vi "testNewArduino.vi"() -> ()   [LabVIEW 2012]
panel:
  in  "valve value":bool
  in  "valve id":i32
  in  "VISA resource":refnum<visa-resource-name>="COM3"
  in  "speed":i32
  in  "Pulse Width in uS":u16(knob)=1300 min=1300 max=2000 step=5 scale=1300.0..2000.0
  in  "servo id":i32=3
  out "light barriers":bool[](array[boolean])
  in  "Stop":bool
  out "loops":i32
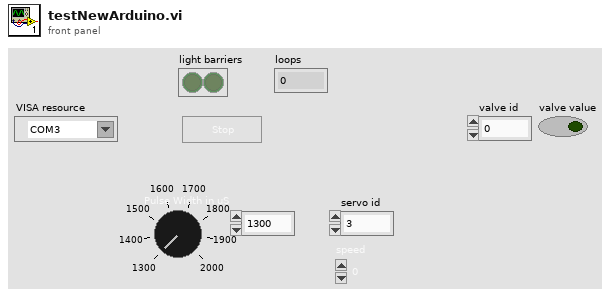
[diagram p1: front panel]
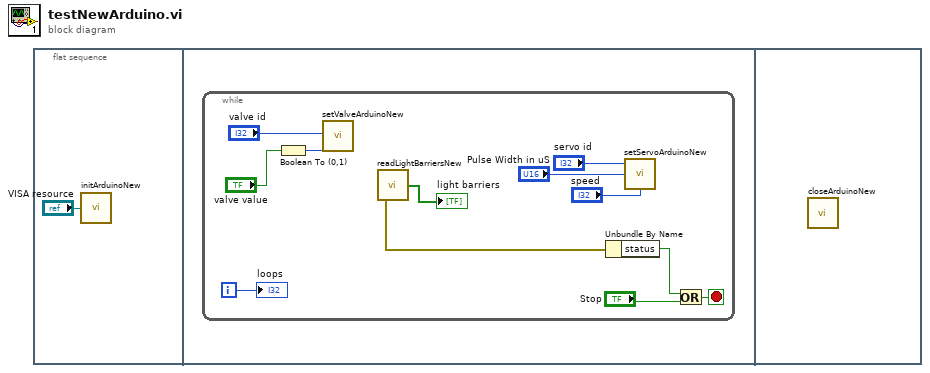
[diagram p0: block diagram]
diagram:
  n1 = flat-sequence {
    frame #0 {
      n2 = call "initArduinoNew.vi"("VISA resource"="VISA resource") -> ()
    }
    frame #1 {
      n3 = while {
        i -> [w10]
        stop <- w13 stop-if-true
        n4 = Boolean To (0,1)(Boolean="valve value") -> (0, 1=w2:i16)
        n5 = call "setValveArduinoNew.vi"("value"=w2, "valve id"="valve id") -> ()  [unwired: 10 in]
        n6 = call "readLightBarriersNew.vi"() -> ("light barriers"=→"light barriers":bool[], "error out"=w8:errorcluster)
        n7 = Unbundle By Name(w8) -> ("status"=w12:bool)
        n8 = call "setServoArduinoNew.vi"("speed"="speed", "Pulse Width in uS"="Pulse Width in uS", "servo id"="servo id") -> ()
        n9 = Or(x=w12, y="Stop") -> (x .or. y?=w13:bool)
        "loops" <- w10
      }
    }
    frame #2 {
      n10 = call "closeArduinoNew.vi"() -> ()  [unwired: 12 in]
    }
  }
